vi "Make Scaling Param Log Input.vi"(0 "String (\"\")":string, 5 "Scaling":T1={"Floating Point Position (2)"=2, "Lower Scaling (1.00E+0)"=0.0, "Upper Scaling (1.00E+2)"=100.0, "Unit Character (\"\")"=""} {"Upper Scaling (1.00E+2)" format="%.2e"; "Lower Scaling (1.00E+0)" format="%.2e"; "Floating Point Position (2)" min=0 max=5 step=1}, 11 "error in (no error)":errorcluster) -> (4 "String After":string, 15 "error out":errorcluster)   [LabVIEW 2020, in "Yokogawa GX Series.lvlib"]
doc: "This VI gets scaling parameter string and concat after input string."
uses:
  <instrlib>/Yokogawa GX Series/Yokogawa GX Series.lvlib
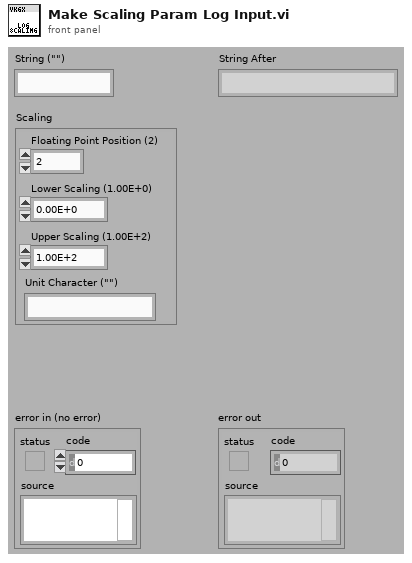
[diagram p1: front panel]
types:
  T1 = cluster{"Floating Point Position (2)":i32, "Lower Scaling (1.00E+0)":dbl, "Upper Scaling (1.00E+2)":dbl, "Unit Character (\"\")":string}
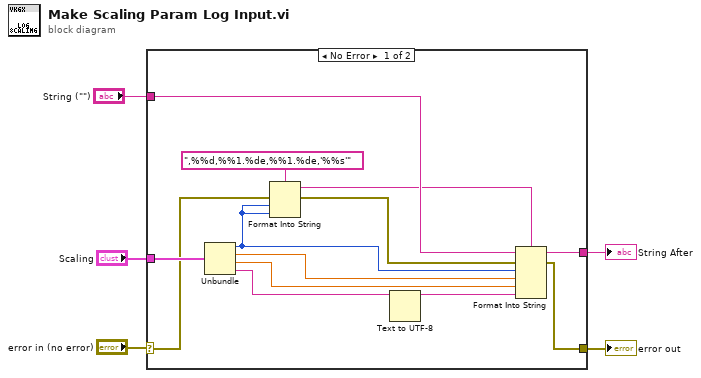
[diagram p0: block diagram]
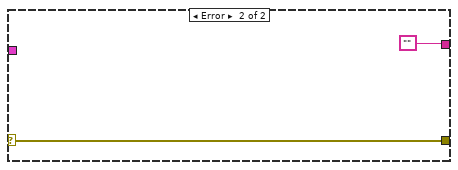
[diagram p2: hidden frame]
diagram:
  n1 = case shown="No Error" "error in (no error)" {
    selector: "error in (no error)" -> [w12 w19]
    tunnel: "Scaling" -> [w18 _]
    tunnel: [w17 ""] -> w4
    tunnel: [w16 w19] -> w3
    tunnel: "String (\"\")" -> [w10 _]
    frame No Error {
      n2 = Unbundle(w18) -> ("Floating Point Position (2)"=w8:i32, "Lower Scaling (1.00E+0)"=w15:dbl, "Upper Scaling (1.00E+2)"=w14:dbl, "Unit Character (\"\")"=w7:string)
      n3 = Format Into String(format string=",%%d,%%1.%de,%%1.%de,'%%s'", error in=w12, w8, w8) -> (resulting string=w9:string, error out=w11:errorcluster)  [unwired: 1 in]
      n4 = Text to UTF-8(11:w7) -> (3:w6:string)  [unwired: 2 in, 1 out]
      n5 = Format Into String(format string=w9, initial string=w10, error in=w11, w8, w15, w14, w6) -> (resulting string=w17:string, error out=w16:errorcluster)
    }
    frame Error {
    }
  }
  "error out" <- w3
  "String After" <- w4
